vi "read_data_rn.vi"(8 "error in (no error)":errorcluster, 11 "RNeighbors in":refnum<class "RNeighbors.lvclass">) -> (0 "error out":errorcluster, 2 "data":T1={"radius"=1.0, "mode"="connectivity", "return_distance"=TRUE, "sort_results"=FALSE}, 3 "RNeighbors out":refnum<class "RNeighbors.lvclass">)   [LabVIEW 2020, in "RNeighbors.lvclass"]
uses:
  RNeighbors.lvclass
  Controls/rneighbors_data.ctl
  RNeighbors.lvclass/RNeighbors.ctl
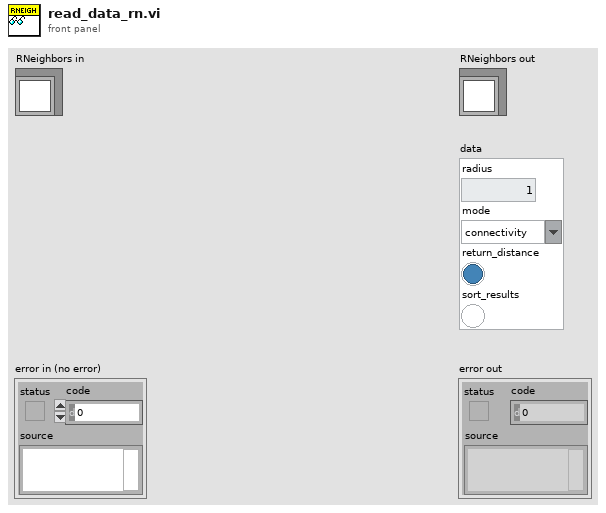
[diagram p1: front panel]
types:
  T1 = typedef "rneighbors_data.ctl" = cluster{"radius":dbl, "mode":string, "return_distance":bool, "sort_results":bool}
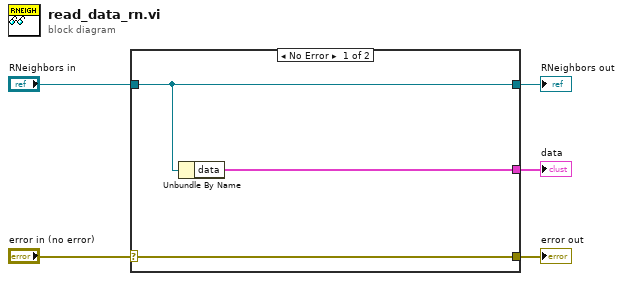
[diagram p0: block diagram]
diagram:
  n1 = case shown="No Error" "error in (no error)" {
    selector: "error in (no error)" -> [w8 w9]
    tunnel: [w8 w9] -> w4
    tunnel: [w7 w10] -> w2
    tunnel: "RNeighbors in" -> [w7 w10]
    tunnel: [w6 _] -> w1
    frame No Error {
      n2 = Unbundle By Name(w7) -> ("data"=w6:T1)
    }
    frame Error {
    }
  }
  "error out" <- w4
  "RNeighbors out" <- w2
  "data" <- w1
